vi "Day 7-2.vi"() -> ()   [LabVIEW 2019, in "Day 7.lvlib"]
uses:
  Day 7.lvlib
panel:
  out "Result":i32
  out "Array":i32[](array[numeric])
  out "array":i32[](array[numeric])
  in  "String":string
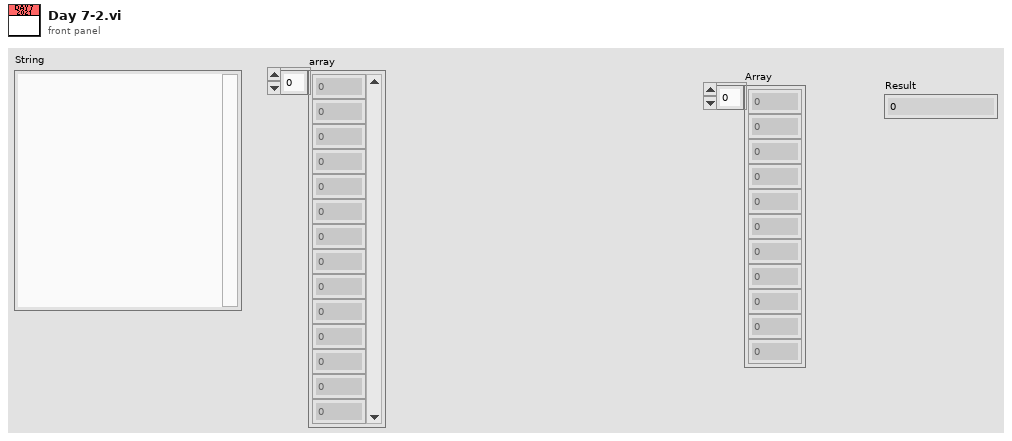
[diagram p1: front panel]
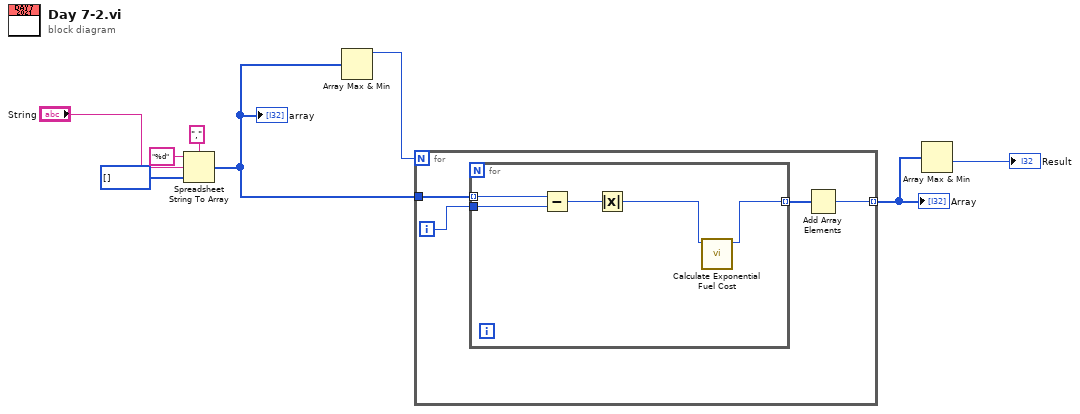
[diagram p0: block diagram]
diagram:
  n1 = Spreadsheet String To Array(delimiter (Tab)=",", format string="%d", spreadsheet string="String", array type (2D Dbl)=i32[] []) -> (array=w4:i32[])
  "array" <- w4
  n2 = Array Max & Min(array=w4) -> (max value=w3:i32)  [unwired: 3 out]
  n3 = for {
    N: w3 -> [_]
    tunnel: w4 -> [w12]
    tunnel: [w10] -> w2 mode=indexing
    i -> [w9]
    n4 = for {
      tunnel: w12 -> [w17] mode=indexing
      tunnel: [w13] -> w11 mode=indexing
      tunnel: w9 -> [w15]
      n5 = Subtract(x=w17, y=w15) -> (x-y=w16:i32)
      n6 = Absolute Value(x=w16) -> (abs(x)=w14:i32)
      n7 = call "Calculate Exponential Fuel Cost.vi"("Numeric"=w14) -> ("Numeric 2"=w13:i32)  [unwired: 10 in]
    }
    n8 = Add Array Elements(numeric array=w11) -> (sum=w10:i32)
  }
  "Array" <- w2
  n9 = Array Max & Min(array=w2) -> (min value=→"Result":i32)  [unwired: 3 out]
